vi "Initialize.vi"(0 "NICal5501 in":refnum<class "Cal Standard.lvclass">, 11 "error in (no error)":errorcluster) -> (4 "NICal5501 out":refnum<class "Cal Standard.lvclass">, 6 "Found":bool, 15 "error out":errorcluster)   [LabVIEW 2023, in "NI Cal-5501 Cal Standard.lvlib" / "Cal Standard.lvclass"]
uses:
  Cal Standard.lvclass
  C:/srd-semi-rfcal-software/AuxTools/STSRFFixtureCharactUtility/Source/Code Modules/Fixture/Instruments/Cal Standard/Cal Standard Base/Cal Standard Base.lvclass
  Cal Standard.lvclass/Cal Standard.ctl
  Instruments/Cal Standard/Cal Standard Base/Cal Standard Base.lvclass/Cal Standard Base.ctl
  Properties/Write Resource Name.vi
  Instruments/Cal Standard/Cal Standard Base/Properties/Write Instrument Info.vi
  Instruments/Cal Standard/Cal Standard Base/Properties/Write Path Connection Map.vi
  Properties/Read Product Name.vi
  <vilib>/nisyscfg/Find Hardware.vi
  <vilib>/nisyscfg/Close (System).vi
  <vilib>/nisyscfg/nisyscfg.lvlib
  <resource>/objmgr/rfSysapiTags.rc
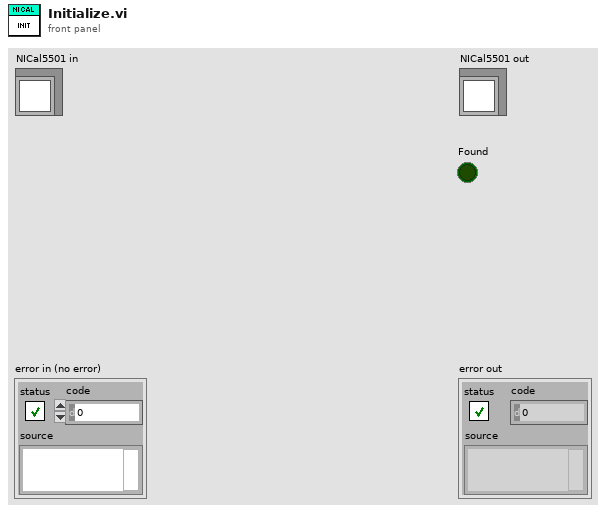
[diagram p1: front panel]
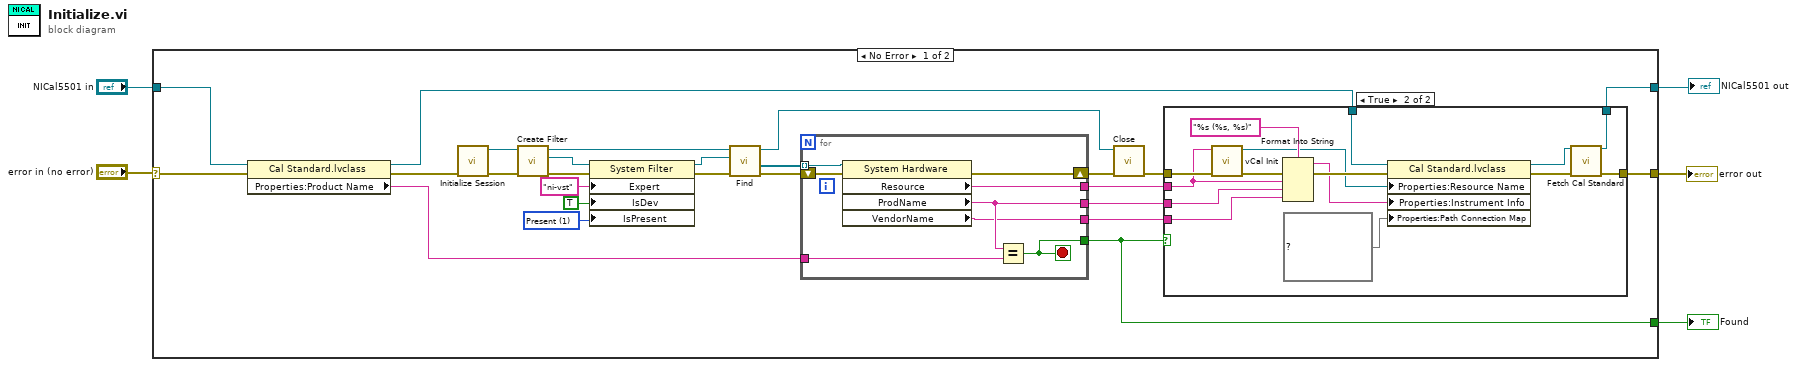
[diagram p0: block diagram]
diagram:
  n1 = case shown="No Error" "error in (no error)" {
    selector: "error in (no error)" -> [w10 w58]
    tunnel: [w15 w58] -> w1
    tunnel: "NICal5501 in" -> [w8 w57]
    tunnel: [w22 w57] -> w3
    tunnel: [w14 _] -> w2
    frame No Error {
      w24 = 1 items=["Unknown"=-1, "Not Present"=0, "Present"=1] ("Devices & Chassis:Is Present")
      n2 = property class="Cal Standard.lvclass"(reference=w8, error in=w10) -> (reference out=w7:refnum<class "Cal Standard.lvclass">, error out=w9:errorcluster, "Properties:Product Name"=w6:string)
      n3 = call <vilib>:"Initialize Session.vi"("error in (no error)"=w9) -> ("error out"=w23:errorcluster, "Session out"=w25:refnum<k21>)  [unwired: 9 in]
      n4 = call <vilib>:"Create Filter.vi"("error in (no error)"=w23, "Session in"=w25) -> ("error out"=w30:errorcluster, "Filter out"=w29:refnum<k20>, "Session out"=w27:refnum<k21>)  [unwired: 7 in]
      n5 = property class="System Filter"(reference=w29, error in=w30, "Expert"="ni-vst" ("Expert Info:Expert Name"), "IsDev"=TRUE ("Is Device"), "IsPresent"=w24) -> (reference out=w28:refnum<k20>, error out=w26:errorcluster)
      n6 = call-poly <vilib>:"Find.vi"("error in (no error)"=w26, "Filter in"=w28, "Session in"=w27) -> ("error out"=w31:errorcluster, "Resources out"=w21:refnum<k20>[], "Session out"=w16:refnum<k21>)  [unwired: 5 in, 1 out]
      n7 = for {
        tunnel: [w53] -> w20
        tunnel: [w54] -> w19
        shift-right: [w55] -> w18
        shift-left: w31 -> [w56]
        tunnel: w21 -> [w52] mode=indexing
        tunnel: [w51] -> w14
        tunnel: [w50] -> w11
        tunnel: w6 -> [w49]
        stop <- w51 stop-if-true
        n8 = property class="System Hardware"(reference=w52, error in=w56) -> (error out=w55:errorcluster, "Resource"=w54:string, "ProdName"=w53:string, "VendorName"=w50:string)  [unwired: 1 out]
        n9 = Equal?(x=w53, y=w49) -> (x = y?=w51:bool)
      }
      n10 = call-poly <vilib>:"Close.vi"("error in (no error)"=w18, "Session in"=w16) -> ("error out"=w17:errorcluster)  [unwired: 9 in]
      n11 = case shown="True" w14 {
        tunnel: w7 -> [w32 w48]
        tunnel: [w32 w35] -> w22
        tunnel: [w33 w36] -> w15
        tunnel: w20 -> [_ w45]
        tunnel: w19 -> [_ w38]
        tunnel: w17 -> [w33 w41]
        tunnel: w11 -> [_ w42]
        frame False {
        }
        frame True {
          n12 = call <instrlib>:"vCal Init.vi"("error in"=w41, "resource name"=w38) -> ("error out"=w40:errorcluster, "instrument handle"=w39:refnum<k15>)  [unwired: 8 in]
          n13 = Format Into String(format string="%s (%s, %s)", error in=w40, w38, w45, w42) -> (resulting string=w44:string, error out=w46:errorcluster)  [unwired: 1 in]
          n14 = property class="Cal Standard.lvclass"(reference=w48, error in=w46, "Properties:Resource Name"=w39, "Properties:Instrument Info"=w44, "Properties:Path Connection Map"=map{string, string[]} {} ("Path Connection Map")) -> (reference out=w34:refnum<class "Cal Standard.lvclass">, error out=w37:errorcluster)
          n15 = call "Fetch Cal Standard.vi"("NICal5501 in"=w34, "error in"=w37) -> ("NICal5501 out"=w35:refnum<class "Cal Standard.lvclass">, "error out"=w36:errorcluster)  [unwired: 12 in]
        }
      }
    }
    frame Error {
    }
  }
  "error out" <- w1
  "NICal5501 out" <- w3
  "Found" <- w2
